vi "PLL.vi"(8 "fc":dbl, 11 "input":dbl) -> (1 "phase":dbl, 3 "frequency":dbl)   [LabVIEW 2016]
panel:
  in  "u3":dbl=0.001
  in  "2*Mu2":dbl=6000.0
  in  "Ts":dbl=3e-06
  in  "2*Mu1":dbl=200.0
  out "sin(phase)":dbl
  out "cos(phase)":dbl
  out "amplitude":dbl
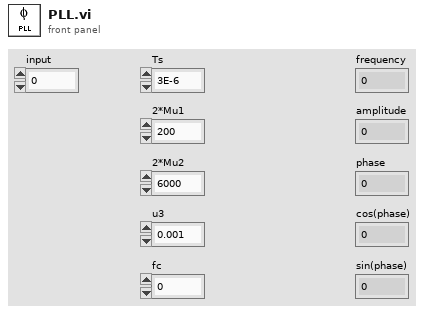
[diagram p1: front panel]
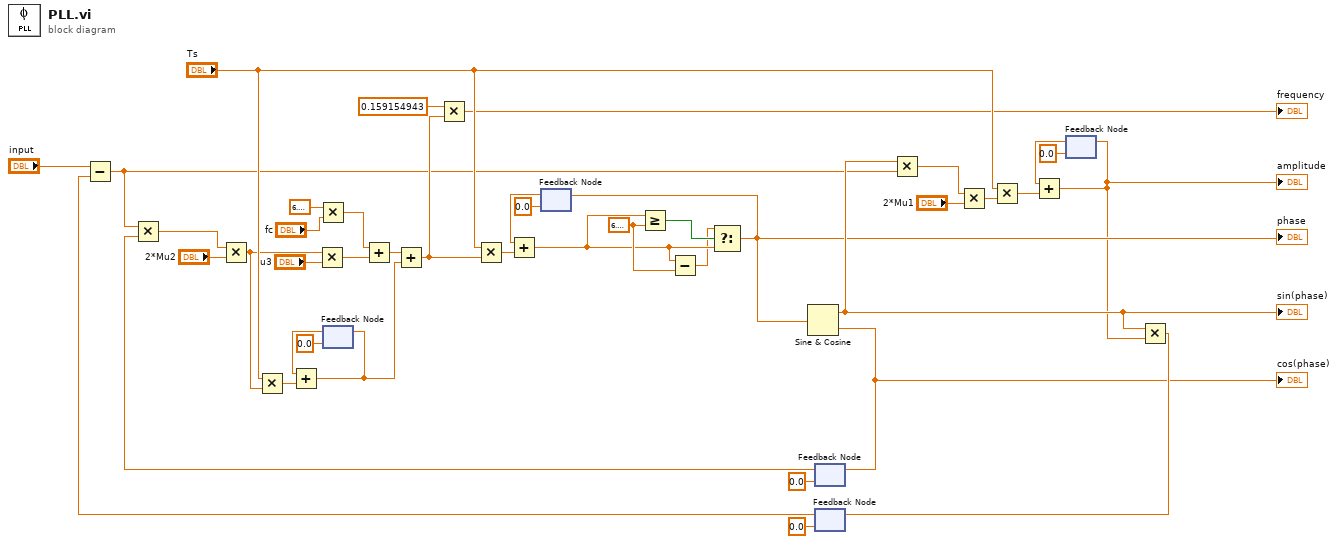
[diagram p0: block diagram]
diagram:
  w12 = 6.283185307179586
  n1 = Multiply(x=6.283185307179586, y="fc") -> (x*y=w22:dbl)
  n2 = feedback #1(0.0) -> (w25:dbl)
  n3 = feedback #2(0.0) -> (w19:dbl)
  n4 = feedback #3(0.0) -> (w30:dbl)
  n5 = feedback #4(0.0) -> (w35:dbl)
  n6 = Subtract(x="input", y=w35) -> (x-y=w3:dbl)
  n7 = Multiply(x=w3, y=w30) -> (x*y=w28:dbl)
  n8 = Multiply(x=w28, y="2*Mu2") -> (x*y=w7:dbl)
  n9 = Multiply(x="Ts", y=w7) -> (x*y=w6:dbl)
  n10 = Add(x=w25, y=w6) -> (x+y=w1:dbl)
  n11 = Multiply(x=w7, y="u3") -> (x*y=w24:dbl)
  n12 = feedback-in #1(w1) -> ()
  n13 = Add(x=w22, y=w24) -> (x+y=w20:dbl)
  n14 = Add(x=w20, y=w1) -> (x+y=w14:dbl)
  n15 = Multiply(x=0.159154943, y=w14) -> (x*y=→"frequency":dbl)
  n16 = Multiply(x="Ts", y=w14) -> (x*y=w13:dbl)
  n17 = Add(x=w19, y=w13) -> (x+y=w9:dbl)
  n18 = Greater Or Equal?(x=w9, y=w12) -> (x >= y?=w11:bool)
  n19 = Subtract(x=w9, y=w12) -> (x-y=w8:dbl)
  n20 = Select(t=w8, s=w11, f=w9) -> (s? t:f=w10:dbl)
  "phase" <- w10
  n21 = feedback-in #2(w10) -> ()
  n22 = Sine & Cosine(0:w10) -> (1:w37:dbl, 2:w31:dbl)
  "cos(phase)" <- w31
  "sin(phase)" <- w37
  n23 = feedback-in #3(w31) -> ()
  n24 = Multiply(x=w37, y=w3) -> (x*y=w39:dbl)
  n25 = Multiply(x=w39, y="2*Mu1") -> (x*y=w2:dbl)
  n26 = Multiply(x="Ts", y=w2) -> (x*y=w4:dbl)
  n27 = feedback #5(0.0) -> (w38:dbl)
  n28 = Add(x=w38, y=w4) -> (x+y=w5:dbl)
  "amplitude" <- w5
  n29 = feedback-in #5(w5) -> ()
  n30 = Multiply(x=w37, y=w5) -> (x*y=w36:dbl)
  n31 = feedback-in #4(w36) -> ()
